vi "New.vi"(6 "Sensor ID":string, 8 "error in (no error)":errorcluster, 9 "Scale Params":dbl[](array[numeric]), 10 "Parent":refnum<class "Config Element.lvclass">, 11 "Scale Type":T1) -> (0 "error out":errorcluster, 3 "Sensor out":refnum<class "Sensor Config.lvclass">)   [LabVIEW 2020, in "VolatusConfig.lvlib" / "Sensor Config.lvclass"]
uses:
  Sensor Config.lvclass
  Sensor Config.lvclass/Sensor Config.ctl
  lv-cdm/CDM-Config/Value Type.ctl
  lv-cdm/CDM-Config/CDM-Config.lvlib
  lv-cdm/CDM-Config/Config Element/Config Element.lvclass
  Scale/Scale Config.lvclass
  VolatusConfigElement/VolatusConfigElement.lvclass
  VolatusConfig.lvlib
  Meta Type.ctl
  C:/dev/lv20CE/relink/lv-volatus/VolatusConfig/VolatusConfigElement/VolatusConfigElement.lvclass
  C:/dev/lv20CE/relink/lv-volatus/VolatusConfig/Sensor/Sensor Config.lvclass
  Scale Type.ctl
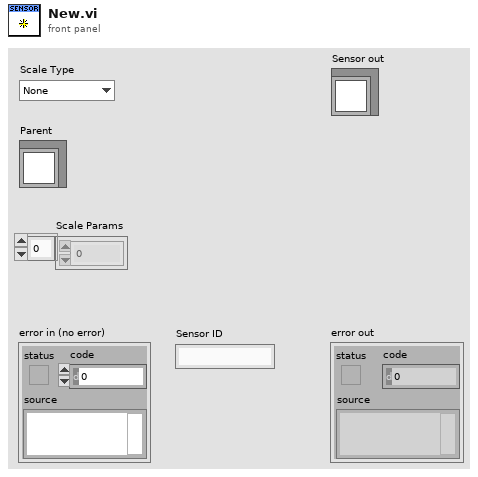
[diagram p1: front panel]
types:
  T1 = typedef "VolatusConfig.lvlib/Scale Type.ctl" = enum16{"None", "Sensor", "Polynomial", "Threshold", "Invert Bool", "Exponential"}
  T2 = typedef "VolatusConfig.lvlib/Meta Type.ctl" = enum16{"UNKNOWN", "VL_System", "VL_Cluster", "VL_Node", "VL_Task", "VL_Group", "VL_Channel", "VL_Task_List", "VL_Scaling", "VL_Sensor", "VL_Sensor_List", "VL_Scale"}
  T3 = typedef "CDM-Config.lvlib/Value Type.ctl" = enum16{"String", "Number", "Bool", "Object", "Array"}
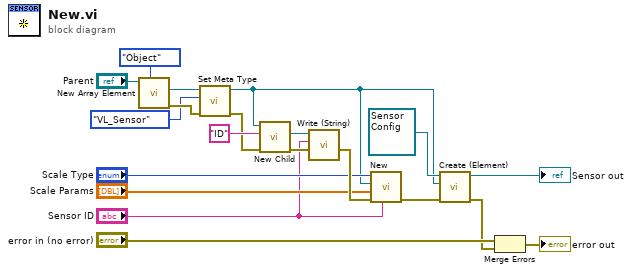
[diagram p0: block diagram]
diagram:
  n1 = call "New Array Element.vi"("Value Type (String)"=Value_Type."Object", "Config Element in"="Parent") -> ("error out"=w16:errorcluster, "New Child"=w4:refnum<class "Config Element.lvclass">)  [unwired: 6 in, 2 out]
  n2 = call "Set Meta Type.vi"("error in (no error)"=w16, "Meta Type"=Meta_Type."VL_Sensor", "Element In"=w4) -> ("error out"=w5:errorcluster, "Element"=w3:refnum<class "Config Element.lvclass">)  [unwired: 7 in]
  n3 = call "New Child.vi"("error in (no error)"=w5, "Child Name"="ID", "Config Element in"=w3) -> ("error out"=w19:errorcluster, "New Child"=w13:refnum<class "Config Element.lvclass">)  [unwired: 6 in, 1 out]
  n4 = call "Write (String).vi"("error in (no error)"=w19, "String Value"="Sensor ID", "Config Element in"=w13) -> ("error out"=w20:errorcluster)  [unwired: 7 in, 1 out]
  n5 = call "New.vi"("Sensor ID (For Sensor Type)"="Sensor ID", "error in (no error)"=w20, "Scale Params (Not Sensor)"="Scale Params", "Parent"=w3, "Scale Type"="Scale Type") -> ("error out"=w8:errorcluster)  [unwired: 5 in, 1 out]
  n6 = call "Create (Element).vi"("error in (no error)"=w8, "Element"=w3, "VolatusConfigElement in"=refnum<class "Sensor Config.lvclass"> refnum ("Sensor in")) -> ("error out"=w6:errorcluster, "VolatusConfigElement out"=→"Sensor out":refnum<class "Sensor Config.lvclass">)  [unwired: 7 in]
  n7 = Merge Errors("error in (no error)", w6) -> (→"error out":errorcluster)
